vi "PGIntialize.vi"(4 "Extra Waits":i32, 5 "On CCD Accumulations":i32=3 min=0 step=1, 6 "Cycle time\n(ms)":i32=3 min=0 step=1, 7 "Number of Frames":i32, 8 "error in":errorcluster, 9 "BIN":u16(ring) items=["1x1", "2x2", "4x4"], 10 "MODE":u16(ring) items=["Normal", "DIF"], 11 "VISA resource name":refnum<visa-resource-name>="COM7") -> (0 "error out":errorcluster, 3 "VISA resource name out":refnum<visa-resource-name>)   [LabVIEW 2018]
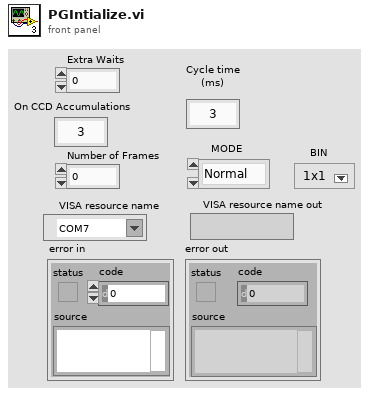
[diagram p1: front panel]
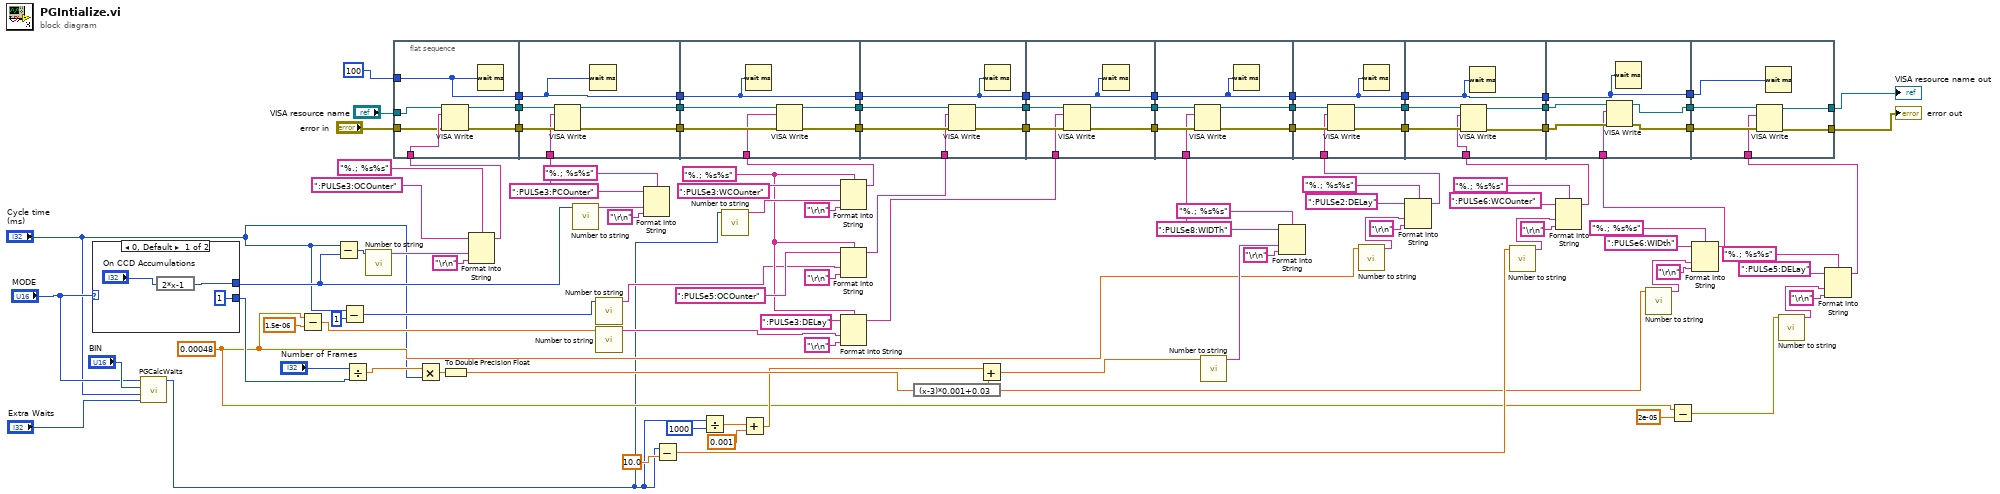
[diagram p0: block diagram]
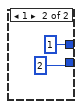
[diagram p2: hidden frame]
diagram:
  w7 = 0.00048
  w66 = "%.; %s%s" ("format string")
  n1 = case shown="0, Default" "MODE" {
    tunnel: [w108 1 ("On CCD Accumulations")] -> w40
    tunnel: [1 ("y") 2 ("On CCD Accumulations")] -> w29
    frame 0, Default {
      n2 = expression code="2*x-1"("On CCD Accumulations") -> (w108:i32)
    }
    frame 1 {
    }
  }
  n3 = call "PGCalcWaits.vi"("Extra Waits"="Extra Waits", "Cycle time\n(ms)"="Cycle time\n(ms)", "BIN"="BIN", "MODE"="MODE") -> ("Wait"=w4:i32)  [unwired: 7 in]
  n4 = Subtract(x=w7, y=1.5e-06) -> (x-y=w56:dbl)
  n5 = Subtract(x="Cycle time\n(ms)", y=w40) -> (x-y=w67:i32)
  n6 = Subtract(x="Cycle time\n(ms)", y=1) -> (x-y=w59:i32)
  n7 = Divide(x="Number of Frames", y=w29) -> (x/y=w30:dbl)
  n8 = call "Number to string.vi"("Numeric"=w67) -> ("Shortest String"=w95:string)  [unwired: 10 in]
  n9 = flat-sequence {
    tunnel: [w118] -> w107
    tunnel: [w117] -> w106
    tunnel: w70 -> [w116]
    tunnel: "error in" -> [w115]
    tunnel: "VISA resource name" -> [w114]
    tunnel: 100 -> [w113]
    tunnel: [w113] -> w27
    tunnel: w107 -> [w124]
    tunnel: w75 -> [w123]
    tunnel: w106 -> [w122]
    tunnel: [w121] -> w105
    tunnel: [w120] -> w104
    tunnel: w27 -> [w119]
    tunnel: [w119] -> w26
    tunnel: w105 -> [w130]
    tunnel: w74 -> [w129]
    tunnel: w104 -> [w128]
    tunnel: [w127] -> w103
    tunnel: [w126] -> w102
    tunnel: w26 -> [w125]
    tunnel: [w125] -> w25
    tunnel: w103 -> [w136]
    tunnel: w73 -> [w135]
    tunnel: w102 -> [w134]
    tunnel: [w133] -> w101
    tunnel: [w132] -> w100
    tunnel: w25 -> [w131]
    tunnel: [w131] -> w24
    tunnel: w101 -> [w142]
    tunnel: w72 -> [w141]
    tunnel: w100 -> [w140]
    tunnel: [w139] -> w99
    tunnel: [w138] -> w98
    tunnel: w24 -> [w137]
    tunnel: [w137] -> w23
    tunnel: w99 -> [w148]
    tunnel: w71 -> [w147]
    tunnel: w98 -> [w146]
    tunnel: [w145] -> w97
    tunnel: [w144] -> w96
    tunnel: w23 -> [w143]
    tunnel: [w143] -> w22
    tunnel: w97 -> [w154]
    tunnel: w62 -> [w153]
    tunnel: w96 -> [w152]
    tunnel: [w151] -> w54
    tunnel: [w150] -> w53
    tunnel: w22 -> [w149]
    tunnel: [w149] -> w21
    tunnel: w54 -> [w160]
    tunnel: w53 -> [w158]
    tunnel: w48 -> [w156]
    tunnel: [w159] -> w47
    tunnel: [w157] -> w46
    tunnel: w21 -> [w155]
    tunnel: [w155] -> w20
    tunnel: w47 -> [w164]
    tunnel: w46 -> [w166]
    tunnel: w42 -> [w162]
    tunnel: w20 -> [w161]
    tunnel: [w163] -> w19
    tunnel: [w165] -> w18
    tunnel: [w161] -> w17
    tunnel: w19 -> [w171]
    tunnel: w18 -> [w170]
    tunnel: w17 -> [w172]
    tunnel: [w169] -> w15
    tunnel: [w168] -> w16
    tunnel: w10 -> [w167]
    frame #0 {
      n10 = VISA Write(VISA resource name=w114, write buffer=w116, error in (no error)=w115) -> (VISA resource name out=w117:refnum<visa-resource-name>, error out=w118:errorcluster)  [unwired: 1 out]
      n11 = Wait (ms)(milliseconds to wait=w113) -> ()  [unwired: 1 out]
    }
    frame #1 {
      n12 = VISA Write(VISA resource name=w122, write buffer=w123, error in (no error)=w124) -> (VISA resource name out=w120:refnum<visa-resource-name>, error out=w121:errorcluster)  [unwired: 1 out]
      n13 = Wait (ms)(milliseconds to wait=w119) -> ()  [unwired: 1 out]
    }
    frame #2 {
      n14 = Wait (ms)(milliseconds to wait=w125) -> ()  [unwired: 1 out]
      n15 = VISA Write(VISA resource name=w128, write buffer=w129, error in (no error)=w130) -> (VISA resource name out=w126:refnum<visa-resource-name>, error out=w127:errorcluster)  [unwired: 1 out]
    }
    frame #3 {
      n16 = VISA Write(VISA resource name=w134, write buffer=w135, error in (no error)=w136) -> (VISA resource name out=w132:refnum<visa-resource-name>, error out=w133:errorcluster)  [unwired: 1 out]
      n17 = Wait (ms)(milliseconds to wait=w131) -> ()  [unwired: 1 out]
    }
    frame #4 {
      n18 = VISA Write(VISA resource name=w140, write buffer=w141, error in (no error)=w142) -> (VISA resource name out=w138:refnum<visa-resource-name>, error out=w139:errorcluster)  [unwired: 1 out]
      n19 = Wait (ms)(milliseconds to wait=w137) -> ()  [unwired: 1 out]
    }
    frame #5 {
      n20 = VISA Write(VISA resource name=w146, write buffer=w147, error in (no error)=w148) -> (VISA resource name out=w144:refnum<visa-resource-name>, error out=w145:errorcluster)  [unwired: 1 out]
      n21 = Wait (ms)(milliseconds to wait=w143) -> ()  [unwired: 1 out]
    }
    frame #6 {
      n22 = VISA Write(VISA resource name=w152, write buffer=w153, error in (no error)=w154) -> (VISA resource name out=w151:refnum<visa-resource-name>, error out=w150:errorcluster)  [unwired: 1 out]
      n23 = Wait (ms)(milliseconds to wait=w149) -> ()  [unwired: 1 out]
    }
    frame #7 {
      n24 = VISA Write(VISA resource name=w160, write buffer=w156, error in (no error)=w158) -> (VISA resource name out=w159:refnum<visa-resource-name>, error out=w157:errorcluster)  [unwired: 1 out]
      n25 = Wait (ms)(milliseconds to wait=w155) -> ()  [unwired: 1 out]
    }
    frame #8 {
      n26 = VISA Write(VISA resource name=w164, write buffer=w162, error in (no error)=w166) -> (VISA resource name out=w163:refnum<visa-resource-name>, error out=w165:errorcluster)  [unwired: 1 out]
      n27 = Wait (ms)(milliseconds to wait=w161) -> ()  [unwired: 1 out]
    }
    frame #9 {
      n28 = VISA Write(VISA resource name=w171, write buffer=w167, error in (no error)=w170) -> (VISA resource name out=w168:refnum<visa-resource-name>, error out=w169:errorcluster)  [unwired: 1 out]
      n29 = Wait (ms)(milliseconds to wait=w172) -> ()  [unwired: 1 out]
    }
  }
  n30 = Multiply(x=w30, y="Cycle time\n(ms)") -> (x*y=w76:dbl)
  n31 = To Double Precision Float(number=w76) -> (double precision float=w41:dbl)
  n32 = Format Into String(format string="%.; %s%s", initial string=":PULSe3:OCOunter" ("format string"), w95, "\r\n" ("format string")) -> (resulting string=w70:string)  [unwired: 1 in, 1 out]
  n33 = call "Number to string.vi"("Numeric"=w40) -> ("Shortest String"=w91:string)  [unwired: 10 in]
  n34 = call "Number to string.vi"("Numeric"=w59) -> ("Shortest String"=w58:string)  [unwired: 10 in]
  n35 = call "Number to string.vi"("Numeric"=w56) -> ("Shortest String"=w55:string)  [unwired: 10 in]
  n36 = Format Into String(format string="%.; %s%s", initial string=":PULSe3:PCOunter" ("format string"), w91, "\r\n" ("format string")) -> (resulting string=w75:string)  [unwired: 1 in, 1 out]
  n37 = Subtract(x=w4, y=10.0) -> (x-y=w38:dbl)
  n38 = Divide(x=w4, y=1000) -> (x/y=w34:dbl)
  n39 = call "Number to string.vi"("Numeric"=w4) -> ("Shortest String"=w81:string)  [unwired: 10 in]
  n40 = Add(x=w34, y=0.001) -> (x+y=w33:dbl)
  n41 = Format Into String(format string=w66, initial string=":PULSe3:WCOunter" ("format string"), w81, "\r\n" ("format string")) -> (resulting string=w74:string)  [unwired: 1 in, 1 out]
  n42 = Format Into String(format string=w66, initial string=":PULSe5:OCOunter" ("format string"), w58, "\r\n" ("format string")) -> (resulting string=w73:string)  [unwired: 1 in, 1 out]
  n43 = Format Into String(format string=w66, initial string=":PULSe3:DELay" ("format string"), w55, "\r\n" ("format string")) -> (resulting string=w72:string)  [unwired: 1 in, 1 out]
  n44 = expression code="(x-3)*0.001+0.03"(w41) -> (w36:dbl)
  n45 = Add(x=w33, y=w36) -> (x+y=w37:dbl)
  n46 = call "Number to string.vi"("Numeric"=w37) -> ("Shortest String"=w78:string)  [unwired: 10 in]
  n47 = Format Into String(format string="%.; %s%s", initial string=":PULSe8:WIDTh" ("format string"), w78, "\r\n" ("format string")) -> (resulting string=w71:string)  [unwired: 1 in, 1 out]
  n48 = call "Number to string.vi"("Numeric"=w7) -> ("Shortest String"=w61:string)  [unwired: 10 in]
  n49 = Format Into String(format string="%.; %s%s", initial string=":PULSe2:DELay" ("format string"), w61, "\r\n" ("format string")) -> (resulting string=w62:string)  [unwired: 1 in, 1 out]
  n50 = call "Number to string.vi"("Numeric"=w38) -> ("Shortest String"=w49:string)  [unwired: 10 in]
  n51 = Format Into String(format string="%.; %s%s", initial string=":PULSe6:WCOunter" ("format string"), w49, "\r\n" ("format string")) -> (resulting string=w48:string)  [unwired: 1 in, 1 out]
  n52 = call "Number to string.vi"("Numeric"=w36) -> ("Shortest String"=w43:string)  [unwired: 10 in]
  n53 = Subtract(x=w7, y=2e-05) -> (x-y=w9:dbl)
  n54 = Format Into String(format string="%.; %s%s", initial string=":PULSe6:WIDth" ("format string"), w43, "\r\n" ("format string")) -> (resulting string=w42:string)  [unwired: 1 in, 1 out]
  n55 = call "Number to string.vi"("Numeric"=w9) -> ("Shortest String"=w11:string)  [unwired: 10 in]
  n56 = Format Into String(format string="%.; %s%s", initial string=":PULSe5:DELay" ("format string"), w11, "\r\n" ("format string")) -> (resulting string=w10:string)  [unwired: 1 in, 1 out]
  "error out" <- w15
  "VISA resource name out" <- w16
